vi "Actor Tree Info.vi"(10 "Actor Data":T1={"Actor Type"="", "Actor Cores"=[], "Self"=refnum, "Caller"=refnum, "Actor Label"="", "Last Ping"=-1.0}) -> (1 "Column Data":string[](array[string]), 2 "Node Name":string, 3 "Parent Tag":string)   [LabVIEW 2017, in "MGI-Monitored Actor.lvlib" / "Classic Monitor.lvclass"]
doc: "Converts the \"Actor Data\" Cluster to tree info\n\nCopyright: MGI 2016\nAuthor: Derek Trepanier"
uses:
  Classic Monitor.lvclass
  monitored-actor-core/Source/Monitor Data/Actor Data.ctl
  <vilib>/ActorFramework/Message Enqueuer/Message Enqueuer.lvclass
  monitored-actor-core/Source/Monitor Data/Monitor Data.lvclass
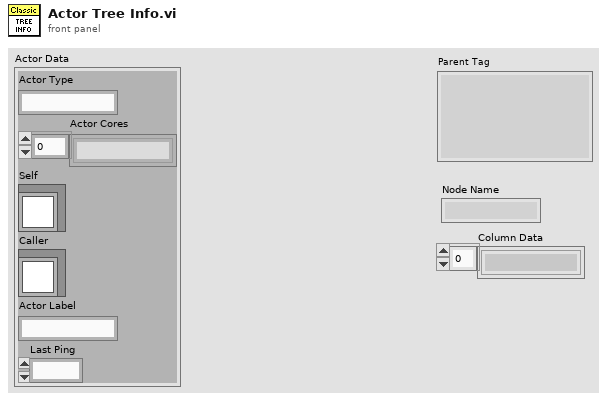
[diagram p1: front panel]
types:
  T1 = typedef "MGI-Monitored Actor Core.lvlib/Monitor Data.lvclass/Actor Data.ctl" = cluster{"Actor Type":string, "Actor Cores":string[], "Self":refnum<class "Message Enqueuer.lvclass">, "Caller":refnum<class "Message Enqueuer.lvclass">, "Actor Label":string, "Last Ping":dbl}
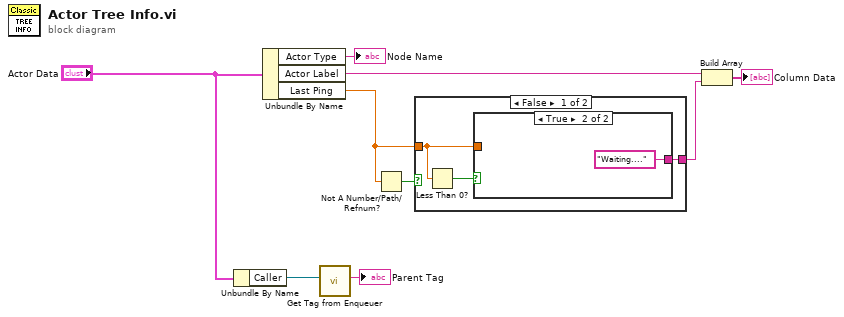
[diagram p0: block diagram]
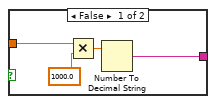
[diagram p2: hidden frame]
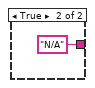
[diagram p3: hidden frame]
diagram:
  n1 = Unbundle By Name("Actor Data") -> ("Caller"=w9:refnum<class "Message Enqueuer.lvclass">)
  n2 = Unbundle By Name("Actor Data") -> ("Actor Type"=→"Node Name":string, "Actor Label"=w8:string, "Last Ping"=w5:dbl)
  n3 = call "Get Tag from Enqueuer.vi"("Enqueuer"=w9) -> ("Tag"=→"Parent Tag":string)  [unwired: 10 in]
  n4 = Not A Number/Path/Refnum?(number/path/refnum=w5) -> (NaN/Path/Refnum?=w6:bool)
  n5 = case shown="False" w6 {
    tunnel: [w12 "N/A"] -> w7
    tunnel: w5 -> [w10 _]
    frame False {
      n6 = Less Than 0?(x=w10) -> (x < 0?=w11:bool)
      n7 = case shown="True" w11 {
        tunnel: [w14 "Waiting...."] -> w12
        tunnel: w10 -> [w13 _]
        frame False {
          n8 = Multiply(x=w13, y=1000.0) -> (x*y=w15:dbl)
          n9 = Number To Decimal String(number=w15) -> (decimal integer string=w14:string)  [unwired: 1 in]
        }
        frame True {
        }
      }
    }
    frame True {
    }
  }
  n10 = Build Array(w8, w7) -> (→"Column Data":string[])
